vi "Interlock.vi"() -> ()   [LabVIEW 2018]
panel:
  out "?":string
  out "?":string
  out "?":string
  out "?":string
  out "?":string
  out "?":string
  out "?":string
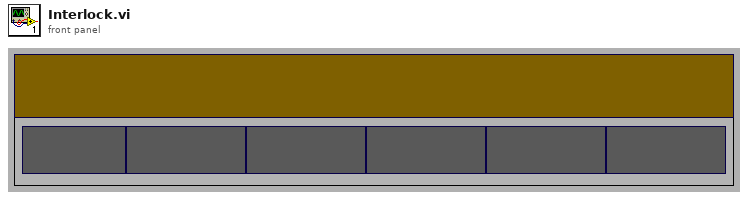
[diagram p1: front panel]
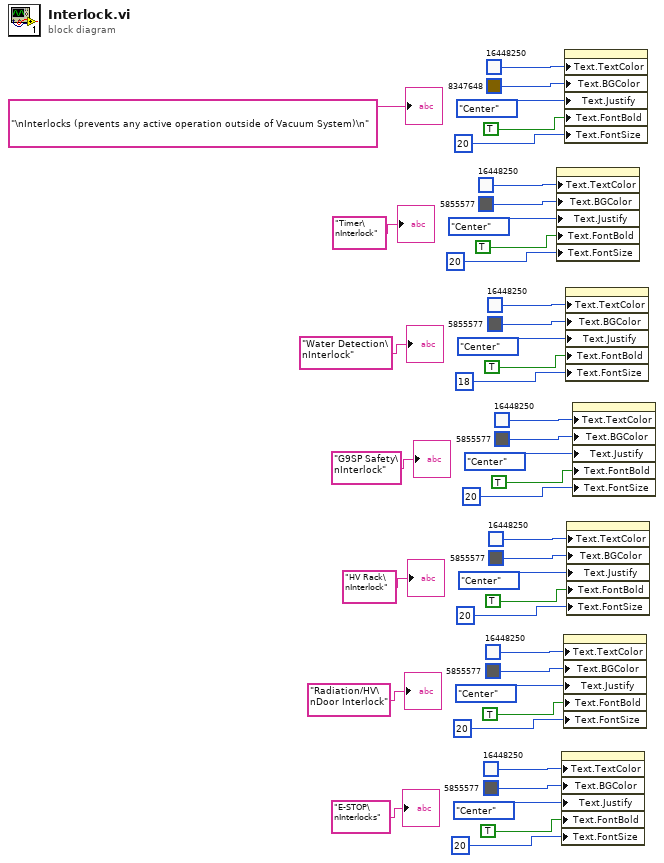
[diagram p0: block diagram]
diagram:
  n1 = property class="Str"("Text.TextColor"=u32 16448250, "Text.BGColor"=u32 5855577, "Text.Justify"=enum16{"Left", "Center", "Right"}."Center" ("Text.Justification"), "Text.FontBold"=TRUE ("Text.Font:Bold"), "Text.FontSize"=u32 20 ("Text.Font:Size")) -> ()  [unwired: 2 in, 2 out]
  n2 = property class="Str"("Text.TextColor"=u32 16448250, "Text.BGColor"=u32 5855577, "Text.Justify"=enum16{"Left", "Center", "Right"}."Center" ("Text.Justification"), "Text.FontBold"=TRUE ("Text.Font:Bold"), "Text.FontSize"=u32 20 ("Text.Font:Size")) -> ()  [unwired: 2 in, 2 out]
  n3 = property class="Str"("Text.TextColor"=u32 16448250, "Text.BGColor"=u32 5855577, "Text.Justify"=enum16{"Left", "Center", "Right"}."Center" ("Text.Justification"), "Text.FontBold"=TRUE ("Text.Font:Bold"), "Text.FontSize"=u32 20 ("Text.Font:Size")) -> ()  [unwired: 2 in, 2 out]
  n4 = property class="Str"("Text.TextColor"=u32 16448250, "Text.BGColor"=u32 8347648, "Text.Justify"=enum16{"Left", "Center", "Right"}."Center" ("Text.Justification"), "Text.FontBold"=TRUE ("Text.Font:Bold"), "Text.FontSize"=u32 20 ("Text.Font:Size")) -> ()  [unwired: 2 in, 2 out]
  n5 = property class="Str"("Text.TextColor"=u32 16448250, "Text.BGColor"=u32 5855577, "Text.Justify"=enum16{"Left", "Center", "Right"}."Center" ("Text.Justification"), "Text.FontBold"=TRUE ("Text.Font:Bold"), "Text.FontSize"=u32 18 ("Text.Font:Size")) -> ()  [unwired: 2 in, 2 out]
  n6 = property class="Str"("Text.TextColor"=u32 16448250, "Text.BGColor"=u32 5855577, "Text.Justify"=enum16{"Left", "Center", "Right"}."Center" ("Text.Justification"), "Text.FontBold"=TRUE ("Text.Font:Bold"), "Text.FontSize"=u32 20 ("Text.Font:Size")) -> ()  [unwired: 2 in, 2 out]
  n7 = property class="Str"("Text.TextColor"=u32 16448250, "Text.BGColor"=u32 5855577, "Text.Justify"=enum16{"Left", "Center", "Right"}."Center" ("Text.Justification"), "Text.FontBold"=TRUE ("Text.Font:Bold"), "Text.FontSize"=u32 20 ("Text.Font:Size")) -> ()  [unwired: 2 in, 2 out]
  "?" <- "\nInterlocks (prevents any active operation outside of Vacuum System)\n" ("String")
  "?" <- "Timer\nInterlock" ("String")
  "?" <- "Water Detection\nInterlock" ("String")
  "?" <- "G9SP Safety\nInterlock" ("String")
  "?" <- "HV Rack\nInterlock" ("String")
  "?" <- "Radiation/HV\nDoor Interlock" ("String")
  "?" <- "E-STOP\nInterlocks" ("String")
